vi "Ensure File Exists.vi"(8 "error in":errorcluster, 10 "Prompt to add new approved file to project?":bool=TRUE, 11 "Approved":path) -> (0 "error out":errorcluster, 3 "File Path":path)   [LabVIEW 2020, in "Approval Tests.lvlib" / "Reporter.lvclass"]
uses:
  Reporter.lvclass
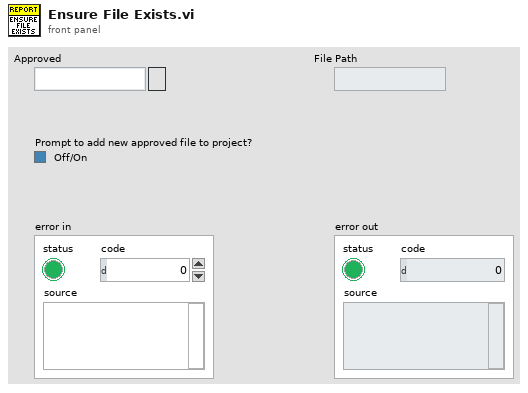
[diagram p1: front panel]
types:
  T1 = enum32{"invalid VI type", "Standard VI", "Control VI", "Global VI", "Polymorphic VI", "Configuration VI", "SubSystem", "Facade VI", "Method VI", "Statechart Diagram VI"}
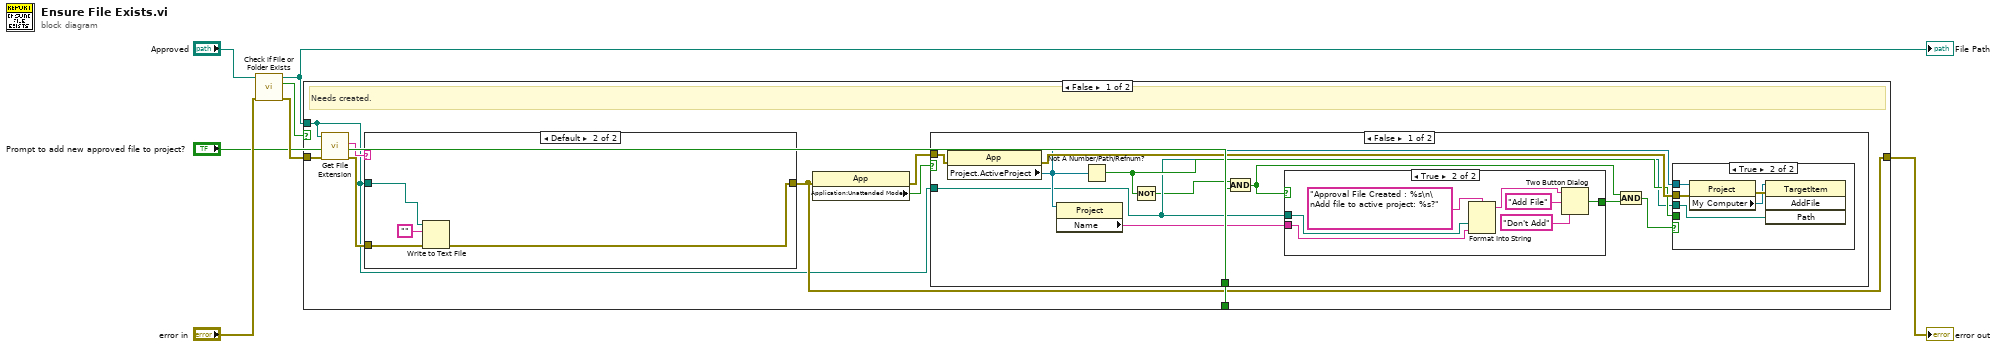
[diagram p0: block diagram]
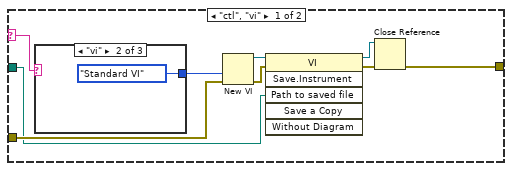
[diagram p5: hidden frame]
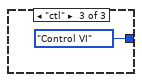
[diagram p7: hidden frame]
diagram:
  n1 = call <vilib>:"Check if File or Folder Exists.vi"("error in (no error)"="error in", "path"="Approved") -> ("error out"=w6:errorcluster, "file or folder exists?"=w3:bool, "dup path"=w2:path)  [unwired: 7 in]
  "File Path" <- w2
  n2 = case shown="False" w3 {
    tunnel: w6 -> [w15 w54]
    tunnel: [w13 w54] -> w5
    tunnel: w2 -> [w9 _]
    tunnel: "Prompt to add new approved file to project?" -> [w8 _]
    frame False {
      # "Needs created."
      n3 = call <vilib>:"Get File Extension.vi"("error in (no error)"=w15, "file"=w9) -> ("error out"=w14:errorcluster, "lowercase file extension"=w11:string)  [unwired: 5 in, 3 out]
      n4 = case shown="Default" w11 {
        selector: w11 -> [w39 _]
        tunnel: [w44 w53] -> w13
        tunnel: w9 -> [w41 w50]
        tunnel: w14 -> [w47 w52]
        frame "ctl", "vi" {
          n5 = case shown="\"vi\"" w39 {
            tunnel: [_ T1."Standard VI" ("vi type (standard vi)") T1."Control VI" ("vi type (standard vi)")] -> w40
            frame Default {
            }
            frame "vi" {
            }
            frame "ctl" {
            }
          }
          n6 = New VI(8:w47, 9:w40) -> (0:w46:errorcluster, 3:w43:refnum<vi>)  [unwired: 5 in]
          n7 = invoke class="VI" method="Save.Instrument"(reference=w43, error in=w46, "Path to saved file"=w41) -> (reference out=w42:refnum<vi>, error out=w45:errorcluster)  [unwired: 3 in, 4 out]
          n8 = Close Reference(reference=w42, error in (no error)=w45) -> (error out=w44:errorcluster)
        }
        frame Default {
          n9 = Write to Text File(file (use dialog)=w50, text="", error in=w52) -> (error out=w53:errorcluster)  [unwired: 1 in, 2 out]
        }
      }
      n10 = property class="App"(error in=w13) -> (error out=w12:errorcluster, "Application:Unattended Mode"=w10:bool)  [unwired: 1 in, 1 out]
      n11 = case shown="False" w10 {
        tunnel: w12 -> [w26 _]
        tunnel: w9 -> [w21 _]
        tunnel: w8 -> [w16 _]
        frame False {
          n12 = property class="App"(error in=w26) -> (error out=w25:errorcluster, "Project.ActiveProject"=w23:refnum<vi>)  [unwired: 1 in, 1 out]
          n13 = property class="Project"(reference=w23) -> ("Name"=w22:string)  [unwired: 1 in, 2 out]
          n14 = Not A Number/Path/Refnum?(number/path/refnum=w23) -> (NaN/Path/Refnum?=w24:bool)
          n15 = Not(x=w24) -> (.not. x?=w18:bool)
          n16 = And(x=w18, y=w16) -> (x .and. y?=w17:bool)
          n17 = case shown="True" w17 {
            tunnel: w22 -> [_ w32]
            tunnel: w21 -> [_ w31]
            tunnel: [_ w30] -> w19
            frame False {
            }
            frame True {
              n18 = Format Into String(format string="Approval File Created : %s\n\nAdd file to active project: %s?", w31, w32) -> (resulting string=w29:string)  [unwired: 2 in, 1 out]
              n19 = Two Button Dialog(message=w29, 1:"Don't Add" ("F button name (\"Cancel\")"), 2:"Add File" ("T button name (\"OK\")")) -> (T button?=w30:bool)
            }
          }
          n20 = And(x=w17, y=w19) -> (x .and. y?=w20:bool)
          n21 = case shown="True" w20 {
            tunnel: w21 -> [_ w36]
            tunnel: w23 -> [_ w35]
            tunnel: w24 -> [_ _]
            tunnel: w25 -> [_ w38]
            frame False {
            }
            frame True {
              n22 = property class="Project"(reference=w35, error in=w38) -> (error out=w37:errorcluster, "My Computer"=w34:refnum<vi>)  [unwired: 1 out]
              n23 = invoke class="TargetItem" method="AddFile"(reference=w34, error in=w37, "Path"=w36) -> ()  [unwired: 1 in, 4 out]
            }
          }
        }
        frame True {
        }
      }
    }
    frame True {
      # "Does exist"
    }
  }
  "error out" <- w5
